vi "Get Server State Ref.vi"(11 "Template Server in":refnum<class "OCV2.lvclass">) -> (2 "Server State Ref":refnum<data-value>, 3 "Template Server out":refnum<class "OCV2.lvclass">)   [LabVIEW 2019, in "OCV2.lvlib" / "OCV2.lvclass"]
uses:
  OCV2.lvclass
  typeDefs/Server State Data.ctl
  OCV2.lvclass/OCV2.ctl
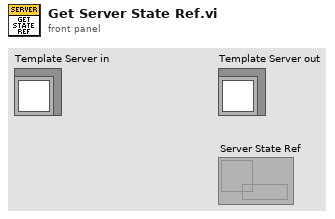
[diagram p1: front panel]
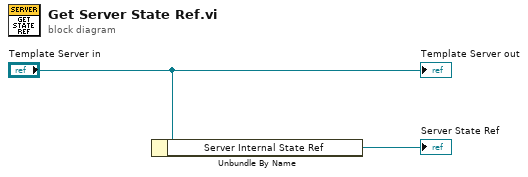
[diagram p0: block diagram]
diagram:
  n1 = Unbundle By Name("Template Server in") -> ("Server Internal State Ref"=→"Server State Ref":refnum<data-value>)
  "Template Server out" <- "Template Server in"
